vi "Controller Average Readings Inputs.vi"(0 "BPM Variables":refnum<k21>[](array[refnum]), 5 "PS Reading Variables":refnum<k21>[](array[refnum]), 7 "PS Status Variables":refnum<k21>[](array[refnum]), 9 "Number of Samples (1000)":dbl=1000.0, 11 "error in (no error)":errorcluster) -> (4 "BPM":dbl[](array[numeric]), 6 "PS":dbl[](array[numeric]), 8 "PS Status (per PS Rack)":u8[](array[numeric]), 15 "error out":errorcluster)   [LabVIEW 2011, in "Controller VIs.lvlib"]
uses:
  Controller VIs.lvlib
  <vilib>/Platform/TimedLoop/XDataNode/timing_clust.ctl
  <vilib>/Platform/TimedLoop/XDataNode/nitl_modes.ctl
  <vilib>/Platform/TimedLoop/XDataNode/wakeup.ctl
  Controller Read FXP20.5.vi
  Controller Read UINT8.vi
  <vilib>/Platform/TimedLoop/XDataNode/loadnilvce.vi
  <vilib>/Platform/TimedLoop/XDataNode/XDataNode.xnode
  <vilib>/Platform/TimedLoop/XDataNode/XDNodeRunTimeDep.lvlib
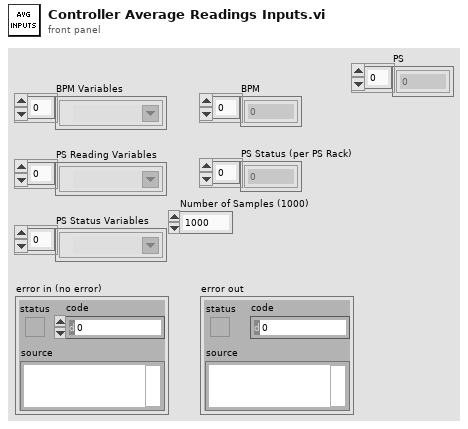
[diagram p1: front panel]
types:
  T1 = typedef "XDNodeRunTimeDep.lvlib/timing_clust.ctl" = cluster{"Expected End [f-1]":u64, "Actual End [f-1]":u64, "Finished Late? [f-1]":bool, "Expected End [i-1]":u64, "Actual End [i-1]":u64, "Finished Late? [i-1]":bool, "Expected Start [i]":u64, "Actual Start [i]":u64, "Expected Start [f]":u64, "Actual Start [f]":u64, "Source Name":string, "Structure Name":string, "Period":i64, "Deadline":i64, "Offset":i64, "Start":i64, "Priority":i32, "Timeout":i32, "Mode":T2, "Wakeup Reason":T3, "Error":errorcluster, "Source Type":string, "Secondary Source Type":string, "Global End Time":u64, "Global Start Time":u64, "Frame Duration":u64, "Iteration Duration":u64, "Assigned CPU":i32, "I/O Scan Engine Mode":u32}
  T2 = typedef "XDNodeRunTimeDep.lvlib/nitl_modes.ctl" = enum32{"No Change", "Process missed periods, maintain original phase", "Discard missed periods, maintain original phase", "Process missed periods, ignore original phase", "Discard missed periods, ignore original phase"}
  T3 = typedef "XDNodeRunTimeDep.lvlib/wakeup.ctl" = enum32{"Normal", "Aborted", "Asynchronous wakeup", "Timing source error", "Timed loop error", "Timeout"}
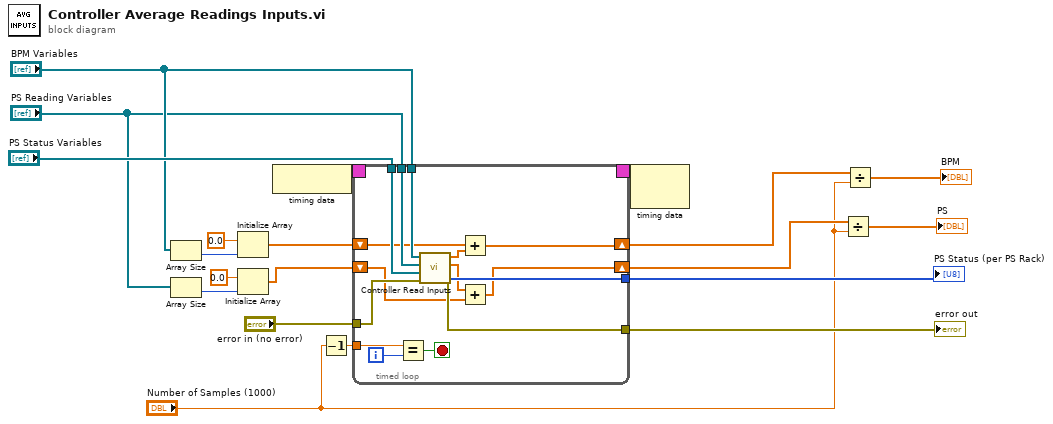
[diagram p0: block diagram]
diagram:
  n1 = Array Size(array="BPM Variables") -> (size(s)=w13:i32)
  n2 = Array Size(array="PS Reading Variables") -> (size(s)=w9:i32)
  n3 = Initialize Array(0.0 ("element"), w13) -> (w11:dbl[])
  n4 = Initialize Array(0.0 ("element"), w9) -> (w8:dbl[])
  n5 = node-c288() -> (w20:T1)
  n6 = Decrement(x="Number of Samples (1000)") -> (x-1=w1:dbl)
  n7 = timed-loop {
    timing: w20 -> [_]
    timing-out: [_] -> w19
    tunnel: [w35] -> w15
    tunnel: "PS Status Variables" -> [w34]
    tunnel: "BPM Variables" -> [w33]
    tunnel: "PS Reading Variables" -> [w32]
    tunnel: [w31] -> w16
    tunnel: "error in (no error)" -> [w30]
    shift-right: [w27] -> w6
    shift-left: w11 -> [w28]
    shift-right: [w26] -> w3
    shift-left: w8 -> [w24]
    tunnel: w1 -> [w21]
    i -> [w23]
    stop <- w22 stop-if-true
    n8 = Equal?(x=w21, y=w23) -> (x = y?=w22:bool)
    n9 = call "Controller Read Inputs.vi"("error in (no error)"=w30, "PS Status Variables"=w34, "PS Reading Variables"=w32, "BPM Variables"=w33) -> ("error out"=w35:errorcluster, "PS Status (per PS Rack)"=w31:u8[], "PS Readings"=w25:dbl[], "BPM Readings"=w29:dbl[])  [unwired: 4 in]
    n10 = Add(x=w28, y=w29) -> (x+y=w27:dbl[])
    n11 = Add(x=w25, y=w24) -> (x+y=w26:dbl[])
  }
  "PS Status (per PS Rack)" <- w16
  "error out" <- w15
  n12 = node-c288(w19) -> ()  [unwired: 1 out]
  n13 = Divide(x=w3, y="Number of Samples (1000)") -> (x/y=→"PS":dbl[])
  n14 = Divide(x=w6, y="Number of Samples (1000)") -> (x/y=→"BPM":dbl[])
